vi "Map (sub vi).vi"() -> (1 "Position":i32[][](array[numeric]), 2 "Display":u32[][](array[colorbox]))   [LabVIEW 2014]
panel:
  in  "Boarder":dbl[][](array[numeric])=[[0.0, 0.0, 18.0, 0.0], [0.0, 1.0, 18.0, 1.0], [0.0, 2.0, 18.0, 2.0], [0.0, 3.0, 18.0, 3.0], [0.0, 4.0, 18.0, 4.0], [0.0, 5.0, 18.0, 5.0], [0.0, 6.0, 18.0, 6.0], [0.0, 7.0, 18.0, 7.0], [0.0, 8.0, 18.0, 8.0], [0.0, 9.0, 18.0, 9.0], [0.0, 10.0, 18.0, 10.0], [0.0, 11.0, 18.0, 11.0], [0.0, 12.0, 18.0, 12.0], [0.0, 13.0, 18.0, 13.0], [0.0, 14.0, 18.0, 14.0], [0.0, 15.0, 18.0, 15.0], [0.0, 16.0, 18.0, 16.0], [0.0, 17.0, 18.0, 17.0], [0.0, 18.0, 18.0, 18.0], [18.0, 0.0, 19.0, 19.0], [18.0, 1.0, 0.0, 0.0], [18.0, 2.0, 0.0, 0.0], [18.0, 3.0, 0.0, 0.0], [18.0, 4.0, 0.0, 0.0], [18.0, 5.0, 0.0, 0.0], [18.0, 6.0, 0.0, 0.0], [18.0, 7.0, 0.0, 0.0], [18.0, 8.0, 0.0, 0.0], [18.0, 9.0, 0.0, 0.0], [18.0, 10.0, 0.0, 0.0], [18.0, 11.0, 0.0, 0.0], [18.0, 12.0, 0.0, 0.0], [18.0, 13.0, 0.0, 0.0], [18.0, 14.0, 0.0, 0.0], [18.0, 15.0, 0.0, 0.0], [18.0, 16.0, 0.0, 0.0], [18.0, 17.0, 0.0, 0.0], [18.0, 18.0, 0.0, 0.0], [0.0, 0.0, 0.0, 0.0], [1.0, 0.0, 0.0, 0.0], [2.0, 0.0, 0.0, 0.0], [3.0, 0.0, 0.0, 0.0], [4.0, 0.0, 0.0, 0.0], [5.0, 0.0, 0.0, 0.0], [6.0, 0.0, 0.0, 0.0], [7.0, 0.0, 0.0, 0.0], [8.0, 0.0, 0.0, 0.0], [9.0, 0.0, 0.0, 0.0], [10.0, 0.0, 0.0, 0.0], [11.0, 0.0, 0.0, 0.0], [12.0, 0.0, 0.0, 0.0], [13.0, 0.0, 0.0, 0.0], [14.0, 0.0, 0.0, 0.0], [15.0, 0.0, 0.0, 0.0], [16.0, 0.0, 0.0, 0.0], [17.0, 0.0, 0.0, 0.0], [18.0, 0.0, 0.0, 0.0], [0.0, 18.0, 0.0, 0.0], [1.0, 18.0, 0.0, 0.0], [2.0, 18.0, 0.0, 0.0], [3.0, 18.0, 0.0, 0.0], [4.0, 18.0, 0.0, 0.0], [5.0, 18.0, 0.0, 0.0], [6.0, 18.0, 0.0, 0.0], [7.0, 18.0, 0.0, 0.0], [8.0, 18.0, 0.0, 0.0], [9.0, 18.0, 0.0, 0.0], [10.0, 18.0, 0.0, 0.0], [11.0, 18.0, 0.0, 0.0], [12.0, 18.0, 0.0, 0.0], [13.0, 18.0, 0.0, 0.0], [14.0, 18.0, 0.0, 0.0], [15.0, 18.0, 0.0, 0.0], [16.0, 18.0, 0.0, 0.0], [17.0, 18.0, 0.0, 0.0], [18.0, 18.0, 0.0, 0.0], [2.0, 2.0, 0.0, 0.0], [2.0, 3.0, 0.0, 0.0], [2.0, 4.0, 0.0, 0.0], [2.0, 5.0, 0.0, 0.0], [2.0, 6.0, 0.0, 0.0], [3.0, 6.0, 0.0, 0.0], [4.0, 6.0, 0.0, 0.0], [4.0, 7.0, 0.0, 0.0], [4.0, 8.0, 0.0, 0.0], [3.0, 8.0, 0.0, 0.0], [2.0, 8.0, 0.0, 0.0], [4.0, 2.0, 0.0, 0.0], [4.0, 3.0, 0.0, 0.0], [4.0, 4.0, 0.0, 0.0], [5.0, 2.0, 0.0, 0.0], [6.0, 2.0, 0.0, 0.0], [7.0, 2.0, 0.0, 0.0], [8.0, 2.0, 0.0, 0.0], [10.0, 1.0, 0.0, 0.0], [10.0, 2.0, 0.0, 0.0], [12.0, 2.0, 0.0, 0.0], [12.0, 3.0, 0.0, 0.0], [13.0, 3.0, 0.0, 0.0], [14.0, 3.0, 0.0, 0.0], [14.0, 1.0, 0.0, 0.0], [16.0, 2.0, 0.0, 0.0], [16.0, 3.0, 0.0, 0.0], [16.0, 4.0, 0.0, 0.0], [16.0, 5.0, 0.0, 0.0], [16.0, 6.0, 0.0, 0.0], [16.0, 7.0, 0.0, 0.0], [14.0, 5.0, 0.0, 0.0], [15.0, 5.0, 0.0, 0.0], [6.0, 4.0, 0.0, 0.0], [7.0, 4.0, 0.0, 0.0], [8.0, 4.0, 0.0, 0.0], [9.0, 4.0, 0.0, 0.0], [10.0, 4.0, 0.0, 0.0], [12.0, 5.0, 0.0, 0.0], [12.0, 6.0, 0.0, 0.0], [12.0, 7.0, 0.0, 0.0], [6.0, 6.0, 0.0, 0.0], [7.0, 6.0, 0.0, 0.0], [8.0, 6.0, 0.0, 0.0], [6.0, 7.0, 0.0, 0.0], [6.0, 8.0, 0.0, 0.0], [8.0, 9.0, 0.0, 0.0], [6.0, 10.0, 0.0, 0.0], [6.0, 11.0, 0.0, 0.0], [6.0, 12.0, 0.0, 0.0], [7.0, 12.0, 0.0, 0.0], [8.0, 12.0, 0.0, 0.0], [10.0, 6.0, 0.0, 0.0], [10.0, 7.0, 0.0, 0.0], [10.0, 8.0, 0.0, 0.0], [10.0, 9.0, 0.0, 0.0], [10.0, 10.0, 0.0, 0.0], [10.0, 11.0, 0.0, 0.0], [10.0, 12.0, 0.0, 0.0], [11.0, 9.0, 0.0, 0.0], [12.0, 9.0, 0.0, 0.0], [14.0, 7.0, 0.0, 0.0], [14.0, 8.0, 0.0, 0.0], [14.0, 9.0, 0.0, 0.0], [14.0, 10.0, 0.0, 0.0], [14.0, 11.0, 0.0, 0.0], [15.0, 9.0, 0.0, 0.0], [16.0, 9.0, 0.0, 0.0], [2.0, 10.0, 0.0, 0.0], [3.0, 10.0, 0.0, 0.0], [4.0, 10.0, 0.0, 0.0], [4.0, 11.0, 0.0, 0.0], [4.0, 12.0, 0.0, 0.0], [3.0, 12.0, 0.0, 0.0], [2.0, 12.0, 0.0, 0.0], [2.0, 13.0, 0.0, 0.0], [2.0, 14.0, 0.0, 0.0], [2.0, 15.0, 0.0, 0.0], [2.0, 16.0, 0.0, 0.0], [4.0, 14.0, 0.0, 0.0], [4.0, 15.0, 0.0, 0.0], [4.0, 16.0, 0.0, 0.0], [5.0, 16.0, 0.0, 0.0], [6.0, 16.0, 0.0, 0.0], [7.0, 16.0, 0.0, 0.0], [8.0, 16.0, 0.0, 0.0], [6.0, 14.0, 0.0, 0.0], [7.0, 14.0, 0.0, 0.0], [8.0, 14.0, 0.0, 0.0], [9.0, 14.0, 0.0, 0.0], [10.0, 14.0, 0.0, 0.0], [10.0, 16.0, 0.0, 0.0], [10.0, 17.0, 0.0, 0.0], [14.0, 17.0, 0.0, 0.0], [12.0, 15.0, 0.0, 0.0], [13.0, 15.0, 0.0, 0.0], [14.0, 15.0, 0.0, 0.0], [12.0, 16.0, 0.0, 0.0], [12.0, 11.0, 0.0, 0.0], [12.0, 12.0, 0.0, 0.0], [12.0, 13.0, 0.0, 0.0], [14.0, 13.0, 0.0, 0.0], [15.0, 13.0, 0.0, 0.0], [16.0, 11.0, 0.0, 0.0], [16.0, 12.0, 0.0, 0.0], [16.0, 13.0, 0.0, 0.0], [16.0, 14.0, 0.0, 0.0], [16.0, 15.0, 0.0, 0.0], [16.0, 16.0, 0.0, 0.0], [8.0, 8.0, 0.0, 0.0], [8.0, 10.0, 0.0, 0.0]]
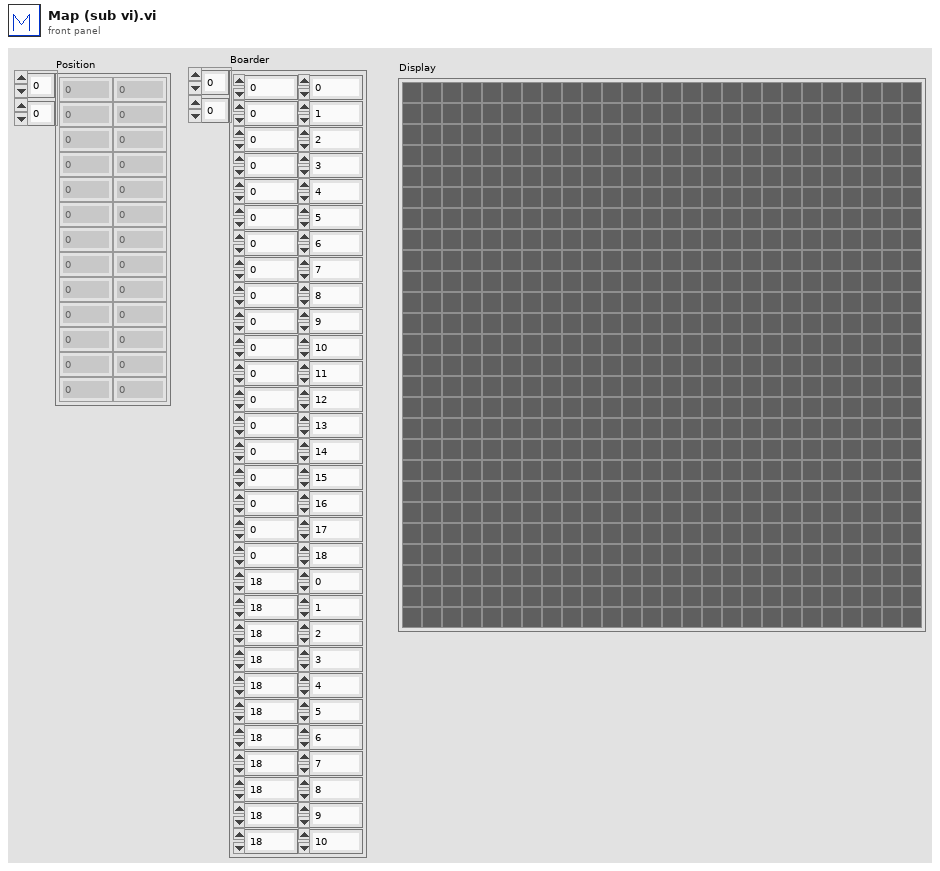
[diagram p1: front panel]
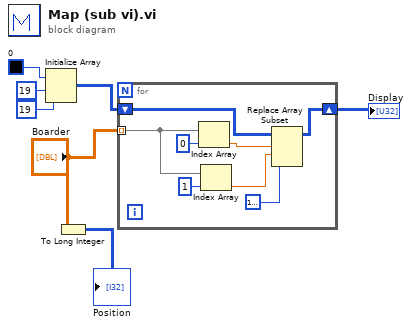
[diagram p0: block diagram]
diagram:
  n1 = Initialize Array(u32 0 ("Color Box"), 19 ("dimension size"), 19 ("dimension size")) -> (w3:u32[][])
  n2 = To Long Integer(number="Boarder") -> (32bit integer=→"Position":i32[][])
  n3 = for {
    tunnel: "Boarder" -> [w8] mode=indexing
    shift-right: [w14] -> w2
    shift-left: w3 -> [w15]
    n4 = Index Array(array=w8, index=0) -> (element=w10:dbl)
    n5 = Index Array(array=w8, index=1) -> (element=w9:dbl)
    n6 = Replace Array Subset(array=w15, new element=u32 16777224 ("Color Box"), index (row)=w10, index (col)=w9) -> (w14:u32[][])
  }
  "Display" <- w2
